vi "CreatePublicEvents.vi"(8 "error in (no error)":errorcluster, 11 "Device":refnum<class "Device.lvclass">) -> (0 "error out":errorcluster, 3 "Device out":refnum<class "Device.lvclass">)   [LabVIEW 2019, in "Device.lvclass"]
doc: "JKI State Machine Objects (SMO) 1.3.0.56\nJKI - JKI\nCopyright (c) 2017, JKI"
uses:
  Device.lvclass
  Typedefs/PublicEvents--Device.Initialized.ctl
  Typedefs/PublicEvents--Device.Uninitialized.ctl
  Device.lvclass/Device.ctl
  <vilib>/JKI/JKI SMO/SMO/SMO.lvclass
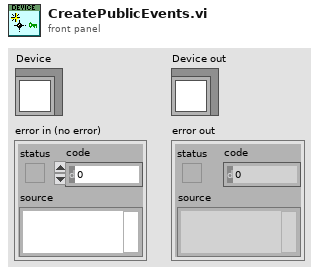
[diagram p1: front panel]
types:
  T1 = typedef "Device.lvclass/PublicEvents--Device.Uninitialized.ctl" = bool
  T2 = typedef "Device.lvclass/PublicEvents--Device.Initialized.ctl" = bool
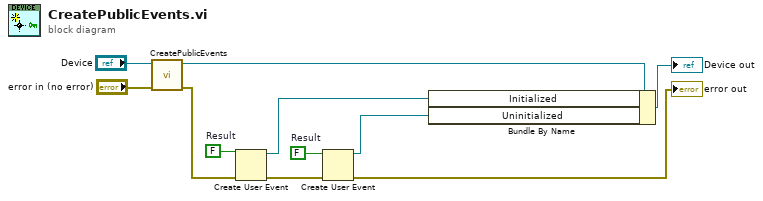
[diagram p0: block diagram]
diagram:
  w4 = T1 FALSE  # Result
  w9 = T2 FALSE  # Result
  n1 = call-parent "CreatePublicEvents.vi"("error in (no error)"="error in (no error)", "SMO"="Device") -> ("error out"=w7:errorcluster, "SMO out"=w8:refnum<class "Device.lvclass">)  [unwired: 8 in]
  n2 = Create User Event(user event datatype=w9, error in=w7) -> (user event=w6:refnum<user-event>, error out=w3:errorcluster)
  n3 = Create User Event(user event datatype=w4, error in=w3) -> (user event=w1:refnum<user-event>, error out=→"error out":errorcluster)
  n4 = Bundle By Name(cluster=w8, "Initialized"=w6, "Uninitialized"=w1) -> (→"Device out":refnum<class "Device.lvclass">)
